vi "set sender.vi"(10 "sender":refnum<class "identifying queue.lvclass">, 11 "message in":refnum<class "communicator message.lvclass">) -> (3 "message out":refnum<class "communicator message.lvclass">)   [LabVIEW 2015, in "communicator message.lvclass"]
uses:
  communicator message.lvclass
  communicator queue/identifying queue.lvclass
  communicator message.lvclass/communicator message.ctl
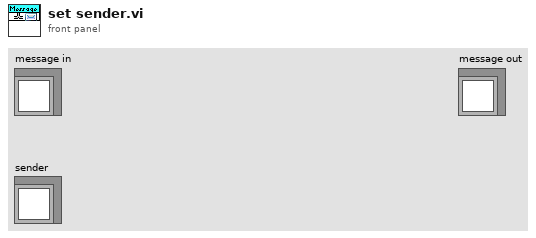
[diagram p1: front panel]
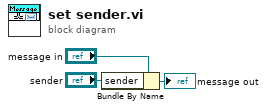
[diagram p0: block diagram]
diagram:
  n1 = Bundle By Name(cluster="message in", "sender"="sender") -> (→"message out":refnum<class "communicator message.lvclass">)
